vi "Configure Timebase.vi"(7 "Record Length (10: 10k points)":u32(ring)=10 items=["1000 points"=1, "10k points"=10, "100k points"=100, "1M points"=1000, "5M points"=5000, "10M points"=10000], 8 "error in (no error)":errorcluster, 9 "Position (10 %)":dbl=10.0, 10 "Timebase (0.0005 s)":dbl=0.0005, 11 "VISA resource name":refnum<visa-resource-name>) -> (0 "error out":errorcluster, 3 "VISA resource name out":refnum<visa-resource-name>)   [LabVIEW 2017, in "Scope.lvlib" / "Tektronix DPO MSO 2000 4000 Series.lvlib"]
doc: "Configures the timebase and horizontal properties of the oscilloscope."
uses:
  Tektronix DPO MSO 2000 4000 Series.lvlib
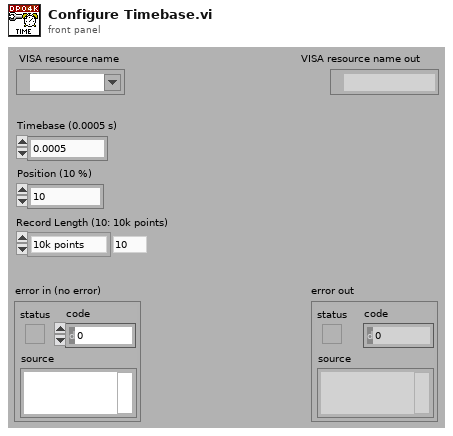
[diagram p1: front panel]
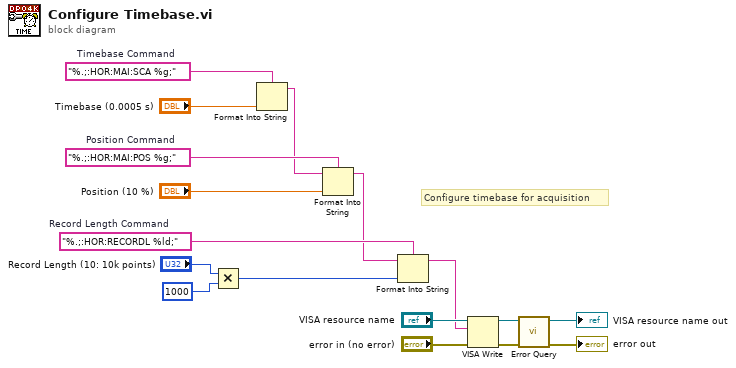
[diagram p0: block diagram]
diagram:
  w7 = "%.;:HOR:RECORDL %ld;"  # Record Length Command
  w10 = "%.;:HOR:MAI:POS %g;"  # Position Command
  w11 = "%.;:HOR:MAI:SCA %g;"  # Timebase Command
  # "Configure timebase for acquisition"
  n1 = Multiply(x="Record Length (10: 10k points)", y=u16 1000) -> (x*y=w4:u32)
  n2 = Format Into String(format string=w11, "Timebase (0.0005 s)") -> (resulting string=w9:string)  [unwired: 2 in, 1 out]
  n3 = Format Into String(format string=w10, initial string=w9, "Position (10 %)") -> (resulting string=w6:string)  [unwired: 1 in, 1 out]
  n4 = Format Into String(format string=w7, initial string=w6, w4) -> (resulting string=w3:string)  [unwired: 1 in, 1 out]
  n5 = VISA Write(VISA resource name="VISA resource name", write buffer=w3, error in (no error)="error in (no error)") -> (VISA resource name out=w13:refnum<visa-resource-name>, error out=w12:errorcluster)  [unwired: 1 out]
  n6 = call "Error Query.vi"("error in (no error)"=w12, "VISA resource name"=w13) -> ("error out"=→"error out":errorcluster, "VISA resource name out"=→"VISA resource name out":refnum<visa-resource-name>)  [unwired: 6 in, 2 out]
